vi "WiiMote Connect by Reference.vi"(8 "error in (no error)":errorcluster, 11 "WiiMote Reference":refnum<k24>) -> (0 "error out":errorcluster, 3 "WiiMote Reference out":refnum<k24>)   [LabVIEW 2012, in "LV Wiimote Interface.lvclass"]
uses:
  LV Wiimote Interface.lvclass
  C:/Program Files/National Instruments/LabVIEW 2012/vi.lib/LabVIEW Hacker/WiiMote/Dependencies/WiimoteLib.dll
  Program Files/National Instruments/LabVIEW 2012/vi.lib/LabVIEW Hacker/WiiMote/Dependencies/WiimoteLib.dll
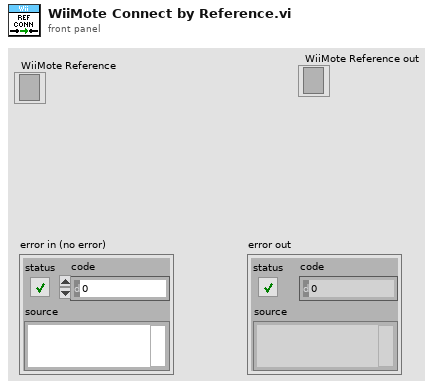
[diagram p1: front panel]
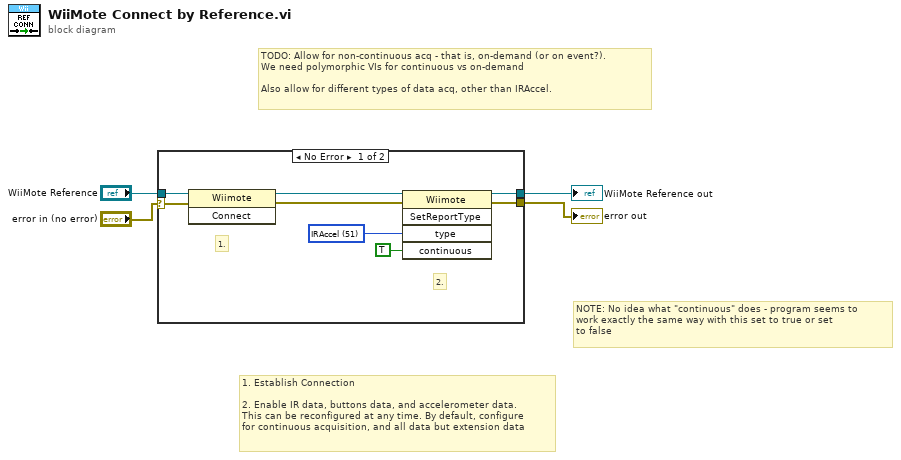
[diagram p0: block diagram]
diagram:
  # "NOTE: No idea what \"continuous\" does - program seems to\nwork exactly the same way with this set to true or set\nto false"
  # "TODO: Allow for non-continuous acq - that is, on-demand (or on event?).\nWe need polymorphic VIs for continuous vs on-demand\n\nAlso allow for different types of data acq, other than IRAccel."
  # "1. Establish Connection\n\n2. Enable IR data, buttons data, and accelerometer data. \nThis can be reconfigured at any time. By default, configure \nfor continuous acquisition, and all data but extension data"
  n1 = case shown="No Error" "error in (no error)" {
    selector: "error in (no error)" -> [w5 w13]
    tunnel: "WiiMote Reference" -> [w9 w14]
    tunnel: [w7 w13] -> w3
    tunnel: [w6 w14] -> w2
    frame No Error {
      w12 = u8 51 items=["Status"=32, "ReadData"=33, "OutputReportAck"=34, "Buttons"=48, "ButtonsAccel"=49, "IRAccel"=51, "ButtonsExtension"=52, "ExtensionAccel"=53, "IRExtensionAccel"=55] ("type")
      # "1."
      # "2."
      n2 = invoke class="Wiimote" method="Connect"(reference=w9, error in=w5) -> (reference out=w11:refnum<k24>, error out=w10:errorcluster)  [unwired: 1 in, 1 out]
      n3 = invoke class="Wiimote" method="SetReportType"(reference=w11, error in=w10, "type"=w12, "continuous"=TRUE) -> (reference out=w6:refnum<k24>, error out=w7:errorcluster)  [unwired: 1 in, 3 out]
    }
    frame Error {
    }
  }
  "error out" <- w3
  "WiiMote Reference out" <- w2
